vi "Do you Keep in Queue.vi"(1 "Queue In":T1(array[cluster])=[{"Measure?"=TRUE, "Area (cm^2)"=0.0, "Cell Label"="", "Cell Description"="", "Cell Position"=0, "Time in rig (h)"=0.0, "Time to next scan (min)"=0.0, "Scan number"=0.0, "When did you stick it in?"=0.0, "Time between scans (min)"=0.0, "Time of the last scan(min)"=0.0, "Scan settings in queue"=0}, {"Measure?"=TRUE, "Area (cm^2)"=0.0, "Cell Label"="", "Cell Description"="", "Cell Position"=0, "Time in rig (h)"=0.0, "Time to next scan (min)"=0.0, "Scan number"=0.0, "When did you stick it in?"=0.0, "Time between scans (min)"=0.0, "Time of the last scan(min)"=0.0, "Scan settings in queue"=0}, {"Measure?"=TRUE, "Area (cm^2)"=0.0, "Cell Label"="", "Cell Description"="", "Cell Position"=0, "Time in rig (h)"=0.0, "Time to next scan (min)"=0.0, "Scan number"=0.0, "When did you stick it in?"=0.0, "Time between scans (min)"=0.0, "Time of the last scan(min)"=0.0, "Scan settings in queue"=0}, {"Measure?"=TRUE, "Area (cm^2)"=0.0, "Cell Label"="", "Cell Description"="", "Cell Position"=0, "Time in rig (h)"=0.0, "Time to next scan (min)"=0.0, "Scan number"=0.0, "When did you stick it in?"=0.0, "Time between scans (min)"=0.0, "Time of the last scan(min)"=0.0, "Scan settings in queue"=0}, {"Measure?"=TRUE, "Area (cm^2)"=0.0, "Cell Label"="", "Cell Description"="", "Cell Position"=0, "Time in rig (h)"=0.0, "Time to next scan (min)"=0.0, "Scan number"=0.0, "When did you stick it in?"=0.0, "Time between scans (min)"=0.0, "Time of the last scan(min)"=0.0, "Scan settings in queue"=0}, {"Measure?"=TRUE, "Area (cm^2)"=0.0, "Cell Label"="", "Cell Description"="", "Cell Position"=0, "Time in rig (h)"=0.0, "Time to next scan (min)"=0.0, "Scan number"=0.0, "When did you stick it in?"=0.0, "Time between scans (min)"=0.0, "Time of the last scan(min)"=0.0, "Scan settings in queue"=0}, {"Measure?"=TRUE, "Area (cm^2)"=0.0, "Cell Label"="", "Cell Description"="", "Cell Position"=0, "Time in rig (h)"=0.0, "Time to next scan (min)"=0.0, "Scan number"=0.0, "When did you stick it in?"=0.0, "Time between scans (min)"=0.0, "Time of the last scan(min)"=0.0, "Scan settings in queue"=0}, {"Measure?"=TRUE, "Area (cm^2)"=0.0, "Cell Label"="", "Cell Description"="", "Cell Position"=0, "Time in rig (h)"=0.0, "Time to next scan (min)"=0.0, "Scan number"=0.0, "When did you stick it in?"=0.0, "Time between scans (min)"=0.0, "Time of the last scan(min)"=0.0, "Scan settings in queue"=0}, {"Measure?"=TRUE, "Area (cm^2)"=0.0, "Cell Label"="", "Cell Description"="", "Cell Position"=0, "Time in rig (h)"=0.0, "Time to next scan (min)"=0.0, "Scan number"=0.0, "When did you stick it in?"=0.0, "Time between scans (min)"=0.0, "Time of the last scan(min)"=0.0, "Scan settings in queue"=0}, {"Measure?"=TRUE, "Area (cm^2)"=0.0, "Cell Label"="", "Cell Description"="", "Cell Position"=0, "Time in rig (h)"=0.0, "Time to next scan (min)"=0.0, "Scan number"=0.0, "When did you stick it in?"=0.0, "Time between scans (min)"=0.0, "Time of the last scan(min)"=0.0, "Scan settings in queue"=0}, {"Measure?"=TRUE, "Area (cm^2)"=0.0, "Cell Label"="", "Cell Description"="", "Cell Position"=0, "Time in rig (h)"=0.0, "Time to next scan (min)"=0.0, "Scan number"=0.0, "When did you stick it in?"=0.0, "Time between scans (min)"=0.0, "Time of the last scan(min)"=0.0, "Scan settings in queue"=0}, {"Measure?"=TRUE, "Area (cm^2)"=0.0, "Cell Label"="", "Cell Description"="", "Cell Position"=0, "Time in rig (h)"=0.0, "Time to next scan (min)"=0.0, "Scan number"=0.0, "When did you stick it in?"=0.0, "Time between scans (min)"=0.0, "Time of the last scan(min)"=0.0, "Scan settings in queue"=0}, {"Measure?"=TRUE, "Area (cm^2)"=0.0, "Cell Label"="", "Cell Description"="", "Cell Position"=0, "Time in rig (h)"=0.0, "Time to next scan (min)"=0.0, "Scan number"=0.0, "When did you stick it in?"=0.0, "Time between scans (min)"=0.0, "Time of the last scan(min)"=0.0, "Scan settings in queue"=0}, {"Measure?"=TRUE, "Area (cm^2)"=0.0, "Cell Label"="", "Cell Description"="", "Cell Position"=0, "Time in rig (h)"=0.0, "Time to next scan (min)"=0.0, "Scan number"=0.0, "When did you stick it in?"=0.0, "Time between scans (min)"=0.0, "Time of the last scan(min)"=0.0, "Scan settings in queue"=0}, {"Measure?"=TRUE, "Area (cm^2)"=0.0, "Cell Label"="", "Cell Description"="", "Cell Position"=0, "Time in rig (h)"=0.0, "Time to next scan (min)"=0.0, "Scan number"=0.0, "When did you stick it in?"=0.0, "Time between scans (min)"=0.0, "Time of the last scan(min)"=0.0, "Scan settings in queue"=0}, {"Measure?"=TRUE, "Area (cm^2)"=0.0, "Cell Label"="", "Cell Description"="", "Cell Position"=0, "Time in rig (h)"=0.0, "Time to next scan (min)"=0.0, "Scan number"=0.0, "When did you stick it in?"=0.0, "Time between scans (min)"=0.0, "Time of the last scan(min)"=0.0, "Scan settings in queue"=0}] {"Scan settings in queue" items=["Regular", "Inverted"]; "Time of the last scan(min)" format="%<%H:%M:%S>t"; "When did you stick it in?" format="%<%H:%M:%S>t"; "Time to next scan (min)" format="%<%H:%M:%S>t"; "Time in rig (h)" format="%<%H:%M:%S>t"}) -> (0 "queue Out":T1(array[cluster])=[{"Measure?"=TRUE, "Area (cm^2)"=0.0, "Cell Label"="", "Cell Description"="", "Cell Position"=0, "Time in rig (h)"=0.0, "Time to next scan (min)"=0.0, "Scan number"=0.0, "When did you stick it in?"=0.0, "Time between scans (min)"=0.0, "Time of the last scan(min)"=0.0, "Scan settings in queue"=0}, {"Measure?"=TRUE, "Area (cm^2)"=0.0, "Cell Label"="", "Cell Description"="", "Cell Position"=0, "Time in rig (h)"=0.0, "Time to next scan (min)"=0.0, "Scan number"=0.0, "When did you stick it in?"=0.0, "Time between scans (min)"=0.0, "Time of the last scan(min)"=0.0, "Scan settings in queue"=0}, {"Measure?"=TRUE, "Area (cm^2)"=0.0, "Cell Label"="", "Cell Description"="", "Cell Position"=0, "Time in rig (h)"=0.0, "Time to next scan (min)"=0.0, "Scan number"=0.0, "When did you stick it in?"=0.0, "Time between scans (min)"=0.0, "Time of the last scan(min)"=0.0, "Scan settings in queue"=0}, {"Measure?"=TRUE, "Area (cm^2)"=0.0, "Cell Label"="", "Cell Description"="", "Cell Position"=0, "Time in rig (h)"=0.0, "Time to next scan (min)"=0.0, "Scan number"=0.0, "When did you stick it in?"=0.0, "Time between scans (min)"=0.0, "Time of the last scan(min)"=0.0, "Scan settings in queue"=0}, {"Measure?"=TRUE, "Area (cm^2)"=0.0, "Cell Label"="", "Cell Description"="", "Cell Position"=0, "Time in rig (h)"=0.0, "Time to next scan (min)"=0.0, "Scan number"=0.0, "When did you stick it in?"=0.0, "Time between scans (min)"=0.0, "Time of the last scan(min)"=0.0, "Scan settings in queue"=0}, {"Measure?"=TRUE, "Area (cm^2)"=0.0, "Cell Label"="", "Cell Description"="", "Cell Position"=0, "Time in rig (h)"=0.0, "Time to next scan (min)"=0.0, "Scan number"=0.0, "When did you stick it in?"=0.0, "Time between scans (min)"=0.0, "Time of the last scan(min)"=0.0, "Scan settings in queue"=0}, {"Measure?"=TRUE, "Area (cm^2)"=0.0, "Cell Label"="", "Cell Description"="", "Cell Position"=0, "Time in rig (h)"=0.0, "Time to next scan (min)"=0.0, "Scan number"=0.0, "When did you stick it in?"=0.0, "Time between scans (min)"=0.0, "Time of the last scan(min)"=0.0, "Scan settings in queue"=0}, {"Measure?"=TRUE, "Area (cm^2)"=0.0, "Cell Label"="", "Cell Description"="", "Cell Position"=0, "Time in rig (h)"=0.0, "Time to next scan (min)"=0.0, "Scan number"=0.0, "When did you stick it in?"=0.0, "Time between scans (min)"=0.0, "Time of the last scan(min)"=0.0, "Scan settings in queue"=0}, {"Measure?"=TRUE, "Area (cm^2)"=0.0, "Cell Label"="", "Cell Description"="", "Cell Position"=0, "Time in rig (h)"=0.0, "Time to next scan (min)"=0.0, "Scan number"=0.0, "When did you stick it in?"=0.0, "Time between scans (min)"=0.0, "Time of the last scan(min)"=0.0, "Scan settings in queue"=0}, {"Measure?"=TRUE, "Area (cm^2)"=0.0, "Cell Label"="", "Cell Description"="", "Cell Position"=0, "Time in rig (h)"=0.0, "Time to next scan (min)"=0.0, "Scan number"=0.0, "When did you stick it in?"=0.0, "Time between scans (min)"=0.0, "Time of the last scan(min)"=0.0, "Scan settings in queue"=0}, {"Measure?"=TRUE, "Area (cm^2)"=0.0, "Cell Label"="", "Cell Description"="", "Cell Position"=0, "Time in rig (h)"=0.0, "Time to next scan (min)"=0.0, "Scan number"=0.0, "When did you stick it in?"=0.0, "Time between scans (min)"=0.0, "Time of the last scan(min)"=0.0, "Scan settings in queue"=0}, {"Measure?"=TRUE, "Area (cm^2)"=0.0, "Cell Label"="", "Cell Description"="", "Cell Position"=0, "Time in rig (h)"=0.0, "Time to next scan (min)"=0.0, "Scan number"=0.0, "When did you stick it in?"=0.0, "Time between scans (min)"=0.0, "Time of the last scan(min)"=0.0, "Scan settings in queue"=0}, {"Measure?"=TRUE, "Area (cm^2)"=0.0, "Cell Label"="", "Cell Description"="", "Cell Position"=0, "Time in rig (h)"=0.0, "Time to next scan (min)"=0.0, "Scan number"=0.0, "When did you stick it in?"=0.0, "Time between scans (min)"=0.0, "Time of the last scan(min)"=0.0, "Scan settings in queue"=0}, {"Measure?"=TRUE, "Area (cm^2)"=0.0, "Cell Label"="", "Cell Description"="", "Cell Position"=0, "Time in rig (h)"=0.0, "Time to next scan (min)"=0.0, "Scan number"=0.0, "When did you stick it in?"=0.0, "Time between scans (min)"=0.0, "Time of the last scan(min)"=0.0, "Scan settings in queue"=0}, {"Measure?"=TRUE, "Area (cm^2)"=0.0, "Cell Label"="", "Cell Description"="", "Cell Position"=0, "Time in rig (h)"=0.0, "Time to next scan (min)"=0.0, "Scan number"=0.0, "When did you stick it in?"=0.0, "Time between scans (min)"=0.0, "Time of the last scan(min)"=0.0, "Scan settings in queue"=0}, {"Measure?"=TRUE, "Area (cm^2)"=0.0, "Cell Label"="", "Cell Description"="", "Cell Position"=0, "Time in rig (h)"=0.0, "Time to next scan (min)"=0.0, "Scan number"=0.0, "When did you stick it in?"=0.0, "Time between scans (min)"=0.0, "Time of the last scan(min)"=0.0, "Scan settings in queue"=0}] {"Scan settings in queue" items=["Regular", "Inverted"]; "Time of the last scan(min)" format="%<%H:%M:%S>t"; "When did you stick it in?" format="%<%H:%M:%S>t"; "Time to next scan (min)" format="%<%H:%M:%S>t"; "Time in rig (h)" format="%<%H:%M:%S>t"})   [LabVIEW 2011]
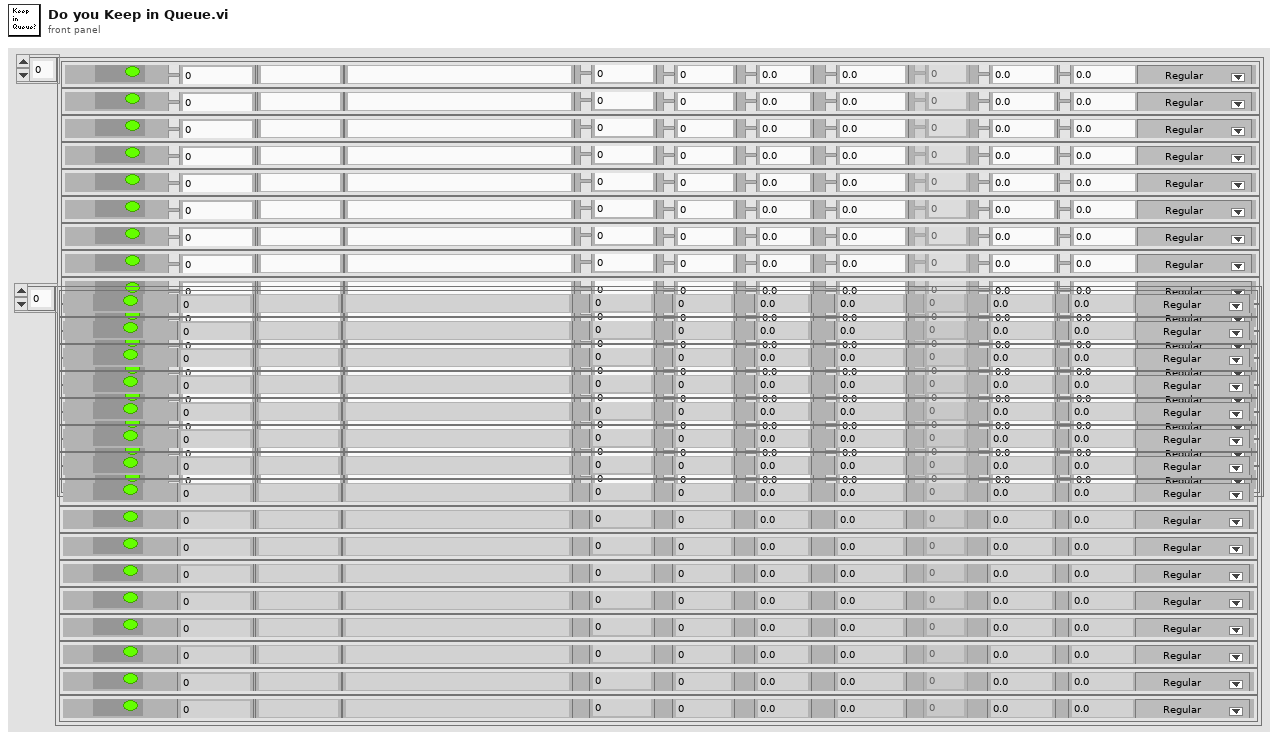
[diagram p1: front panel]
types:
  T1 = cluster{"Measure?":bool, "Area (cm^2)":dbl, "Cell Label":string, "Cell Description":string, "Cell Position":i32, "Time in rig (h)":dbl, "Time to next scan (min)":dbl, "Scan number":dbl, "When did you stick it in?":dbl, "Time between scans (min)":dbl, "Time of the last scan(min)":dbl, "Scan settings in queue":u16}[]
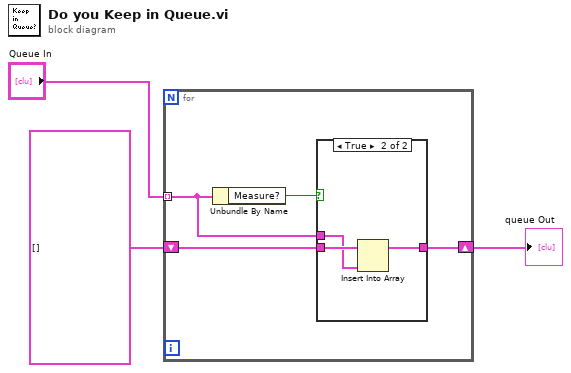
[diagram p0: block diagram]
diagram:
  n1 = for {
    shift-right: [w7] -> w1
    shift-left: T1 [] ("Queue In") -> [w6]
    tunnel: "Queue In" -> [w4] mode=indexing
    n2 = Unbundle By Name(w4) -> ("Measure?"=w5:bool)
    n3 = case shown="True" w5 {
      tunnel: [w8 w9] -> w7
      tunnel: w6 -> [w8 w11]
      tunnel: w4 -> [_ w10]
      frame False {
      }
      frame True {
        n4 = Insert Into Array(array=w11, new element=w10) -> (w9:T1)  [unwired: 1 in]
      }
    }
  }
  "queue Out" <- w1
